vi "Robot Center Indicator.vi"(8 "error in (no error)":errorcluster) -> (0 "error out":errorcluster, 3 "Robot Center":i32=80)   [LabVIEW 2016]
uses:
  Robot Global Data.vi
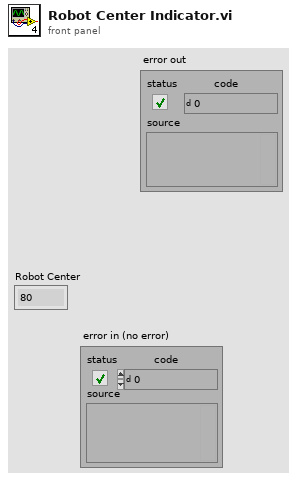
[diagram p1: front panel]
types:
  T1 = typedef "WPI_CameraImageSize.ctl" = enum16{"640x480", "320x240", "160x120", "Custom"}
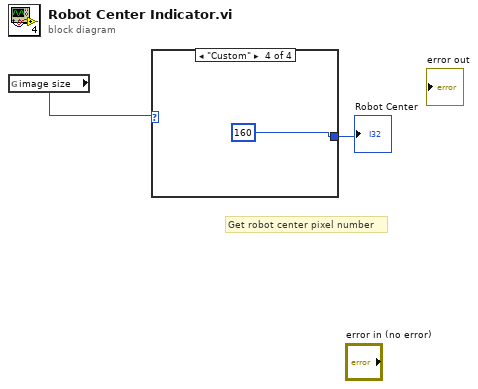
[diagram p0: block diagram]
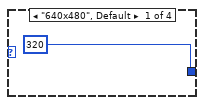
[diagram p2: hidden frame]
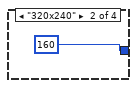
[diagram p3: hidden frame]
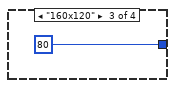
[diagram p4: hidden frame]
diagram:
  # "Get robot center pixel number"
  n1 = global read "Robot Global Data.vi" "image size"() -> (w2:T1)
  n2 = case shown="\"Custom\"" w2 {
    tunnel: [320 160 80 160] -> w1
    frame "640x480", Default {
    }
    frame "320x240" {
    }
    frame "160x120" {
    }
    frame "Custom" {
    }
  }
  "Robot Center" <- w1
